vi "习题4.3.vi"() -> ()   [LabVIEW 2018]
panel:
  out "数值":dbl
  in  "x":dbl
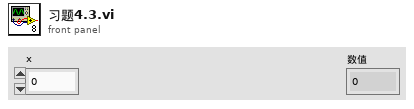
[diagram p1: front panel]
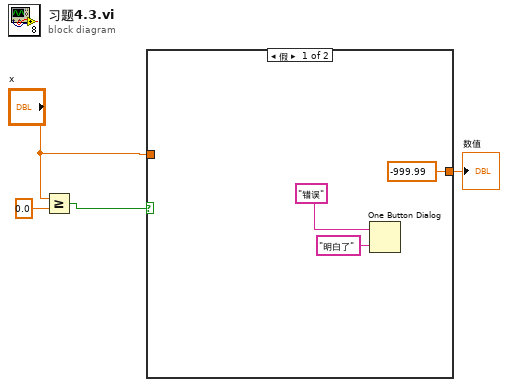
[diagram p0: block diagram]
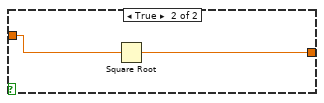
[diagram p2: hidden frame]
diagram:
  n1 = Greater Or Equal?(x="x", y=0.0) -> (x >= y?=w4:bool)
  n2 = case shown="假" w4 {
    tunnel: "x" -> [_ w9]
    tunnel: [-999.99 w8] -> w1
    frame False {
      n3 = One Button Dialog(message="错误", button name ("OK")="明白了" ("按钮名称（“确定”）")) -> ()  [unwired: 1 out]
    }
    frame True {
      n4 = Square Root(x=w9) -> (sqrt(x)=w8:dbl)
    }
  }
  "数值" <- w1
